vi "Calibration_Warning.vi"(11 "USB":tag) -> ()   [LabVIEW 2015]
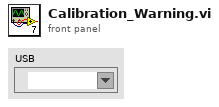
[diagram p1: front panel]
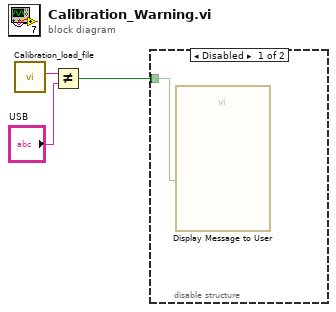
[diagram p0: block diagram]
diagram:
  n1 = call "Calibration_load_file.vi"() -> ("USB_DEV"=w2:string)  [unwired: 10 in, 1 out]
  n2 = Not Equal?(x=w2, y="USB") -> (x != y?=w1:bool)
  n3 = disable-structure shown="Disabled" {
    disable-tunnel: w1 -> [w4 _]
    frame Disabled {
      n4 = call "Display Message to User"("Enable"=w4) -> ()  [unwired: 9 in, 2 out]
    }
    frame Enabled {
    }
  }
